vi "set led.vi"(8 "error in (no error)":errorcluster, 10 "led":T1(ring), 11 "index":i32) -> (0 "error out":errorcluster)   [LabVIEW 2017, in "libfreenect.lvlib"]
doc: "EXPORT void freenect_lv_set_led(freenect_led_options led, int index);"
uses:
  libfreenect.lvlib
  freenect_lv.dll
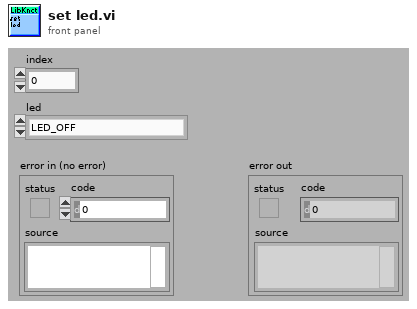
[diagram p1: front panel]
types:
  T1 = enum16{"LED_OFF", "LED_GREEN", "LED_RED", "LED_YELLOW", "LED_BLINK_GREEN", "LED_BLINK_GREEN2", "LED_BLINK_RED_YELLOW"}
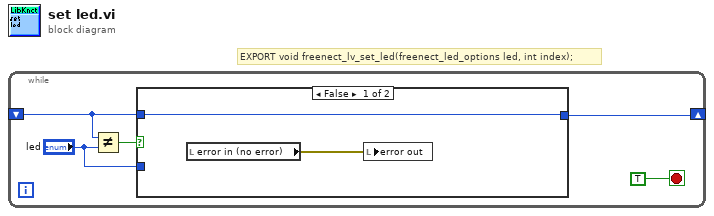
[diagram p0: block diagram]
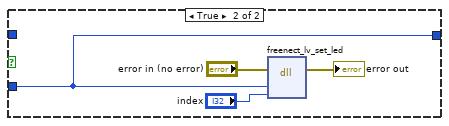
[diagram p2: hidden frame]
diagram:
  # "EXPORT void freenect_lv_set_led(freenect_led_options led, int index);"
  n1 = while {
    shift-right: [w1] -> _
    shift-left: _ -> [w3]
    stop <- TRUE stop-if-true
    n2 = Not Equal?(x=w3, y="led") -> (x != y?=w4:bool)
    n3 = case shown="False" w4 {
      tunnel: [w7 w8] -> w1
      tunnel: w3 -> [w7 _]
      tunnel: "led" -> [_ w8]
      frame False {
        n4 = local read "error in (no error)"() -> (w6:errorcluster)
        n5 = local write "error out"(w6) -> ()
      }
      frame True {
        n6 = dll-call lib="C:/Users/Mats/Desktop/Bacheler prosjekt/Labview/Occupancy Grid Map Code - With model/freenect_lv.*" fn="freenect_lv_set_led"(error in="error in (no error)", "led"=w8, "index"="index") -> (error out=→"error out":errorcluster)  [unwired: 3 in, 3 out]
      }
    }
  }
